vi "convertor imagine.vi"() -> ()   [LabVIEW 2024]
uses:
  <vilib>/vision/NI_Vision_Development_Module.lvlib
panel:
  out "Image":T1(plugin-control)
  out "appended path":path
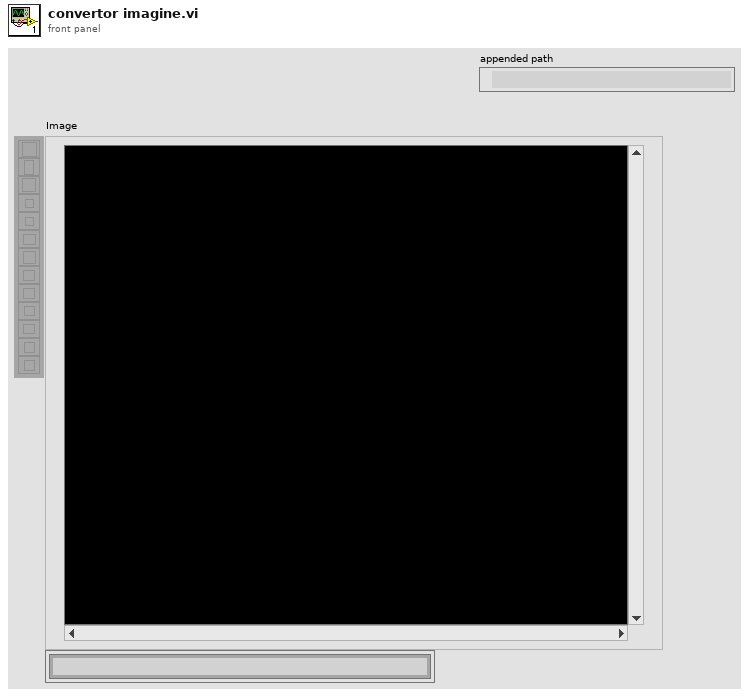
[diagram p1: front panel]
types:
  T1 = typedef "IMAQ Image.ctl" = refnum<image>
  T2 = typedef "Image Type" = u32
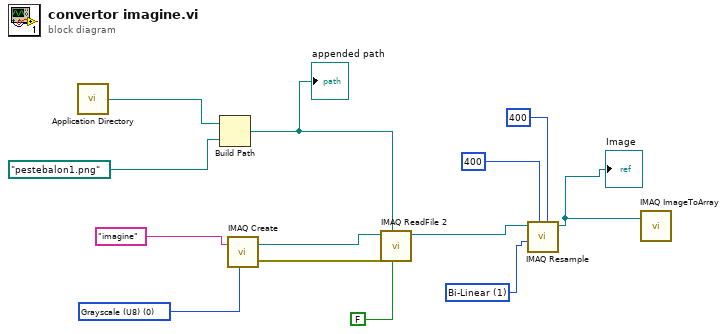
[diagram p0: block diagram]
diagram:
  w10 = u32 1 items=["Zero Order", "Bi-Linear", "Quadratic", "Cubic Spline"] ("Interpolation Type")
  w12 = T2 0 items=["Grayscale (U8)", "Grayscale (I16)", "Grayscale (SGL)", "Complex (CSG)", "RGB (U32)", "HSL (U32)", "RGB (U64)", "Grayscale (U16)"] ("Image Type")
  n1 = call <vilib>:"Application Directory.vi"() -> ("Application Directory"=w3:path)
  n2 = Build Path(base path=w3, name or relative path=path "pestebalon1.png" ("File Path")) -> (appended path=w5:path)
  "appended path" <- w5
  n3 = call "IMAQ Create"("Image Name"="imagine", "Image Type"=w12) -> ("New Image"=w2:T1, "error out"=w11:errorcluster)  [unwired: 3 in]
  n4 = call "IMAQ ReadFile 2"("Use File Path Image Type"=FALSE, "File Path"=w5, "error in (no error)"=w11, "Image"=w2) -> ("Image Out"=w9:T1)  [unwired: 3 in, 4 out]
  n5 = call "IMAQ Resample"("X Resolution"=400, "Y Resolution"=400, "Interpolation Type"=w10, "Image Src"=w9) -> ("Image Dst Out"=w1:T1)  [unwired: 6 in, 1 out]
  "Image" <- w1
  n6 = call "IMAQ ImageToArray"("Image"=w1) -> ()  [unwired: 3 in, 5 out]
